vi "P3AT_Panel_Msg.vi"(8 "error in (no error)":errorcluster caption="错误输入（无错误）", 10 "值(信号)":T1={"max_vel"=0.49056603773584906, "max_rot"=0.5094339622641509, "Control_Mode"=enum."Joy"} {"max_rot" scale=0.0..1.0; "max_vel" scale=0.0..1.0}, 11 "CoordinatorState输入":refnum<class "CoordinatorState.lvclass">) -> (0 "error out":errorcluster caption="错误输出", 3 "Process State out":refnum<class "State Actor.lvclass">)   [LabVIEW 2014, in "States.lvlib" / "CoordinatorState.lvclass"]
uses:
  CoordinatorState.lvclass
  ctl/P3AT_Panel.ctl
  <vilib>/NI/Actors/State Actor/State Actor/State Actor.lvclass
  ctl/P3AT_Current.ctl
  CoordinatorState.lvclass/CoordinatorState.ctl
  <vilib>/ActorFramework/Message Enqueuer/Message Enqueuer.lvclass/Message Enqueuer.ctl
  <vilib>/ActorFramework/Message Enqueuer/Enqueue.vi
  Global_var/Global_var.vi
  <vilib>/ActorFramework/Message Priority Queue/Priority Enqueue.vi
  Process State Messages/Go to Running Msg/Go to Voice Msg.lvclass
  Process State Messages/Go to Idle Msg/Go to Ready Msg.lvclass
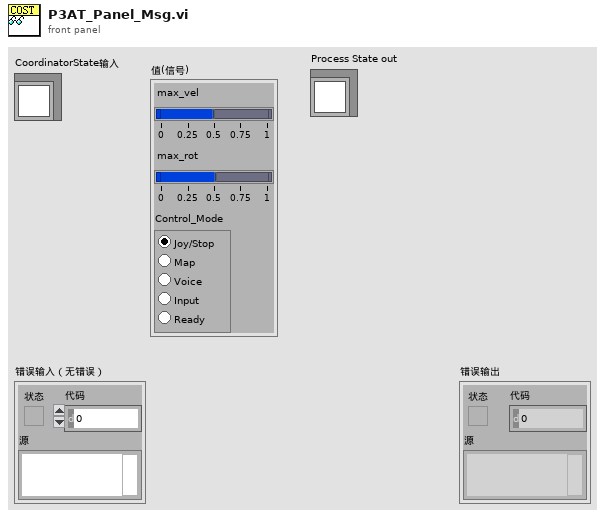
[diagram p1: front panel]
types:
  T1 = typedef "P3AT_Panel.ctl" = cluster{"max_vel":dbl, "max_rot":dbl, "Control_Mode":enum32{"Joy", "Map", "Voice", "Input", "Undefined"}}
  T2 = typedef "P3AT_Current.ctl" = cluster{"max_vel":dbl, "max_rot":dbl, "now_pose_X":dbl, "now_pose_Y":dbl, "now_pose_Rot_deg":dbl, "Control_Mode":enum32{"Joy", "Map", "Voice", "Input", "Undefined"}}
  T3 = enum32{"Joy", "Map", "Voice", "Input", "Undefined"}
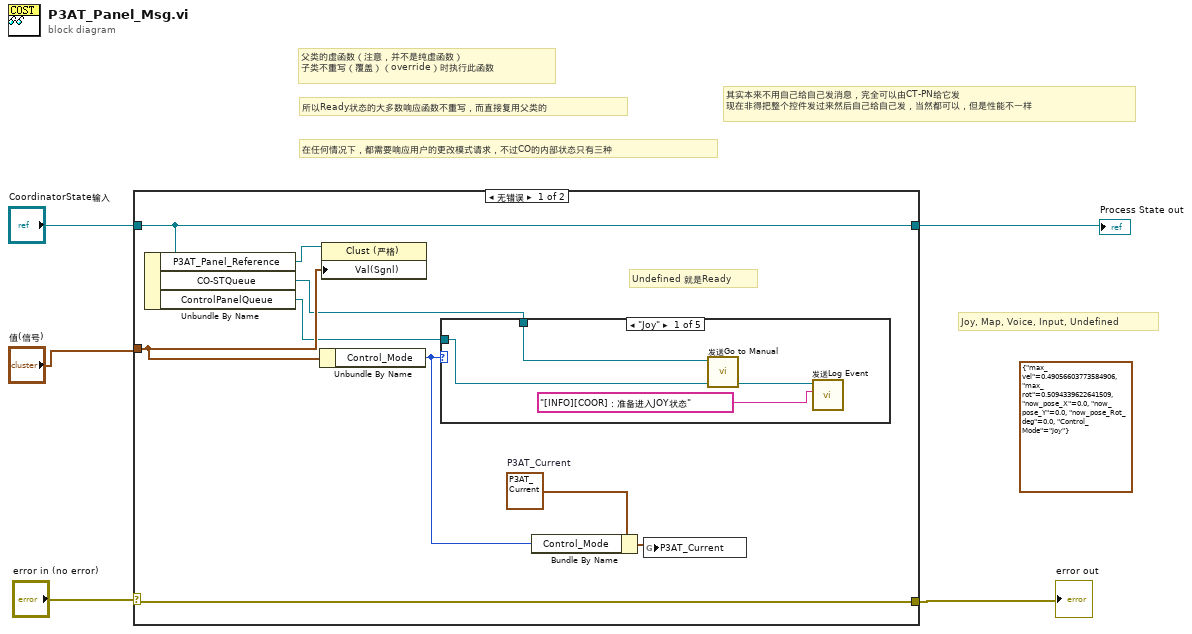
[diagram p0: block diagram]
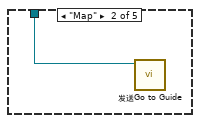
[diagram p2: hidden frame]
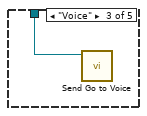
[diagram p3: hidden frame]
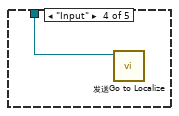
[diagram p4: hidden frame]
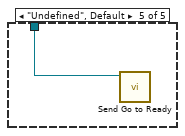
[diagram p5: hidden frame]
diagram:
  (unwired) T2 {"max_vel"=0.49056603773584906, "max_rot"=0.5094339622641509, "now_pose_X"=0.0, "now_pose_Y"=0.0, "now_pose_Rot_deg"=0.0, "Control_Mode"=enum."Joy"} ("P3AT_Current")
  # "Joy, Map, Voice, Input, Undefined"
  # "其实本来不用自己给自己发消息，完全可以由CT-PN给它发\n现在非得把整个控件发过来然后自己给自己发，当然都可以，但是性能不一样"
  # "所以Ready状态的大多数响应函数不重写，而直接复用父类的"
  # "在任何情况下，都需要响应用户的更改模式请求，不过CO的内部状态只有三种"
  # "父类的虚函数（注意，并不是纯虚函数）\n子类不重写（覆盖）（override）时执行此函数"
  n1 = case shown="无错误" "error in (no error)" {
    selector: "error in (no error)" -> [w14 w22]
    tunnel: [w14 w22] -> w4
    tunnel: [w10 w23] -> w1
    tunnel: "CoordinatorState输入" -> [w10 w23]
    tunnel: "值(信号)" -> [w12 _]
    frame No Error {
      w9 = T2 {"max_vel"=0.49056603773584906, "max_rot"=0.5094339622641509, "now_pose_X"=0.0, "now_pose_Y"=0.0, "now_pose_Rot_deg"=0.0, "Control_Mode"=enum."Joy"}  # P3AT_Current
      # "Undefined 就是Ready"
      n2 = Unbundle By Name(w10) -> ("P3AT_Panel_Reference"=w13:refnum<vi>, "CO-STQueue"=w11:refnum<class "Message Enqueuer.lvclass">, "ControlPanelQueue"=w6:refnum<class "Message Enqueuer.lvclass">)
      n3 = Unbundle By Name(w12) -> ("Control_Mode"=w7:T3)
      n4 = property class="Clust (严格)"(reference=w13, "Val(Sgnl)"=w12) -> ()  [unwired: 1 in, 2 out]
      n5 = case shown="\"Joy\"" w7 {
        tunnel: w11 -> [w17 w18 w19 w20 w21]
        tunnel: w6 -> [w16 _ _ _ _]
        frame "Joy" {
          n6 = call "发送Go to Manual.vi"("消息待入队列"=w17) -> ()  [unwired: 9 in, 2 out]
          n7 = call "发送Log Event.vi"("Event Text"="[INFO][COOR]：准备进入JOY状态", "消息待入队列"=w16) -> ()  [unwired: 8 in, 2 out]
        }
        frame "Map" {
          n8 = call "发送Go to Guide.vi"("消息待入队列"=w18) -> ()  [unwired: 9 in, 2 out]
        }
        frame "Voice" {
          n9 = call "Send Go to Voice.vi"("Message Enqueuer"=w19) -> ()  [unwired: 9 in, 2 out]
        }
        frame "Input" {
          n10 = call "发送Go to Localize.vi"("消息待入队列"=w20) -> ()  [unwired: 9 in, 2 out]
        }
        frame "Undefined", Default {
          n11 = call "Send Go to Ready.vi"("Message Enqueuer"=w21) -> ()  [unwired: 9 in, 2 out]
        }
      }
      n12 = Bundle By Name(cluster=w9, "Control_Mode"=w7) -> (w8:T2)
      n13 = global write "Global_var.vi" "P3AT_Current"(w8) -> ()
    }
    frame Error {
    }
  }
  "error out" <- w4
  "Process State out" <- w1
